vi "Handle Event.vi"(8 "error in (no error)":errorcluster, 9 "Event Source in":refnum<class "Event Source.lvclass">, 10 "Event Data":refnum<class "Event.lvclass">, 11 "Update Boolean Msg in":refnum<class "Update Boolean Msg.lvclass">) -> (0 "error out":errorcluster, 1 "Event Source out":refnum<class "Event Source.lvclass">, 3 "Update Boolean Msg out":refnum<class "Update Boolean Msg.lvclass">)   [LabVIEW 2016, in "Example Source.lvlib" / "Update Boolean Msg.lvclass"]
uses:
  Update Boolean Msg.lvclass
  Example Source/Example Source.lvclass
  Example Events/Boolean Event.lvclass
  C:/Projects/Shared Libraries/Event Actors/Event Source/Event Source.lvclass
  Event Source/Event Source.lvclass
  Event/Event.lvclass
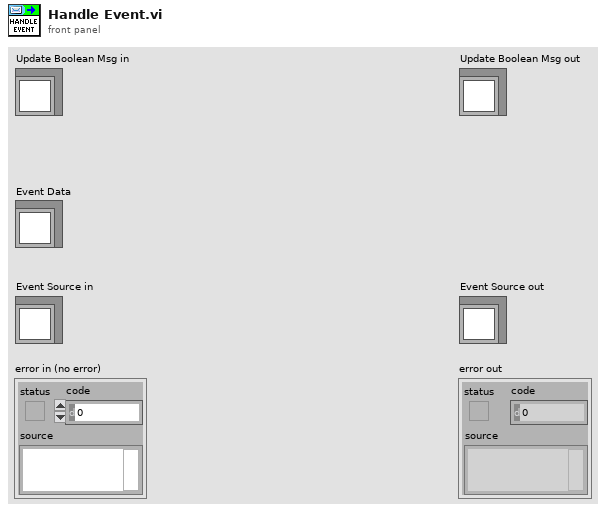
[diagram p1: front panel]
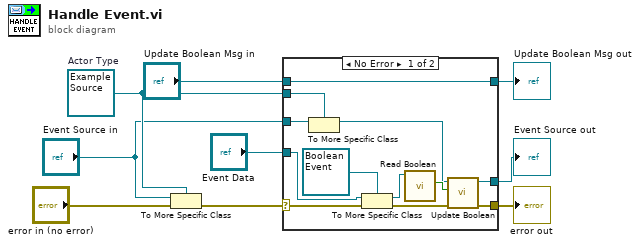
[diagram p0: block diagram]
diagram:
  w8 = refnum<class "Example Source.lvclass"> refnum  # Actor Type
  n1 = To More Specific Class(target class=w8, reference="Event Source in", error in="error in (no error)") -> (error out=w9:errorcluster)  [unwired: 1 out]
  n2 = case shown="No Error" w9 {
    selector: w9 -> [w16 w23]
    tunnel: "Event Source in" -> [w13 w24]
    tunnel: "Update Boolean Msg in" -> [w10 w22]
    tunnel: [w17 w23] -> w1
    tunnel: w8 -> [w14 _]
    tunnel: [w12 w24] -> w3
    tunnel: "Event Data" -> [w11 _]
    tunnel: [w10 w22] -> w5
    frame No Error {
      n3 = To More Specific Class(target class=w14, reference=w13) -> (specific class reference=w15:refnum<class "Example Source.lvclass">)  [unwired: 1 in, 1 out]
      n4 = To More Specific Class(target class=refnum<class "Boolean Event.lvclass"> refnum ("Example Source.lvlib:Boolean Event.lvclass"), reference=w11, error in=w16) -> (specific class reference=w19:refnum<class "Boolean Event.lvclass">, error out=w18:errorcluster)
      n5 = call "Read Boolean.vi"("Double Array Event in"=w19) -> ("Boolean"=w20:bool)  [unwired: 9 in, 1 out]
      n6 = call "Update Boolean.vi"("error in (no error)"=w18, "Boolean"=w20, "Example Source in"=w15) -> ("error out"=w17:errorcluster, "Example Source out"=w12:refnum<class "Example Source.lvclass">)  [unwired: 7 in]
    }
    frame Error {
    }
  }
  "error out" <- w1
  "Update Boolean Msg out" <- w5
  "Event Source out" <- w3
